vi "PH_gentec_M-Link.constructor.vi"(0 "name":string, 2 "data in":string, 5 "error in":errorcluster) -> (14 "i ref out":refnum<vi>, 16 "data out":string, 19 "error out":errorcluster)   [LabVIEW 2014, in "PH_gentec_M-Link.lvlib"]
doc: "This class is forseen to control a gentec-M-Link Energy- or Powermeter.\n\nThis class is part of the PHELIX device layer.\n\nauthor: Stefan Götte, GSI\n\nLicense Agreement for this software:\n\nCopyright (C)\nGesellschaft für Schwerionenforschung, GSI\nPlanckstr. 1\n64291 Darmstadt\nGermany\n\nContact: D.Beck@gsi.de \n\nThis program is free software; you can redistribute it and/or modify it under the terms of the \nGNU General Public License as published by the Free Software Foundation; either version 2 of \nthe license, or (at your option) any later version.\n\nThis program is distributed in the hope that it will be useful, but WITHOUT ANY WARRANTY; \nwithout even the implied warranty of MERCHANTABILITY or FITNESS FOR A PARTICULAR PURPOSE. See the GNU General License for more details (http://www.gnu.org).\n\nGesellschaft für Schwerionenforschung, GSI\nPlanckstr. 1, 64291 Darmstadt, Germany\nFor all questions and ideas contact: M.Richter@gsi.de, H.Brand@gsi.de or D.Beck@gsi.de.\nLast update: 16-JUN-2004"
uses:
  PH_gentec_M-Link.lvlib
  PH_Basics/PH_Powermeter_BaseClass/PH_Powermeter_BaseClass.State.ctl
  PH_Basics/PH_Class/PH_Class.lvlib
  PH_Basics/PH_Powermeter_BaseClass/PH_Powermeter_BaseClass.lvlib
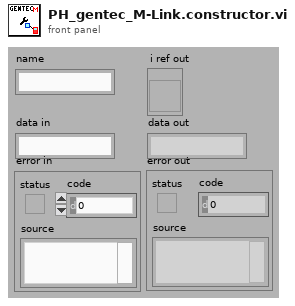
[diagram p1: front panel]
types:
  T1 = typedef "PH_Powermeter_BaseClass.lvlib/PH_Powermeter_BaseClass.State.ctl" = enum32{"off", "operating", "opened", "checked", "connected", "Sets to change", "running"}
  T2 = enum16{"SetAttribute", "GetAttribute", "CreateAttribute", "DestroyAttribute", "DestroyAllAtributes"}
  T3 = typedef "PH_gentec_M-Link.lvlib/PH_gentec_M-Link.i attribute.ctl" = cluster{"GUI References":cluster{"Wanted Head Settings":refnum<vi>, "Current Head Settings":refnum<vi>, "Set Auto Range":refnum<vi>, "Trigger Polarity":refnum<vi>, "Trigger Source":refnum<vi>, "Waveform Averages":refnum<vi>, "Continuous":refnum<vi>, "get one Value":refnum<vi>}, "Wanted Head Settings":T4, "Current Head Settings":T4}
  T4 = typedef "PH_gentec_M-Link.lvlib/PH_gentec_M-Link.Head Settings.ctl" = cluster{"Measurement Mode":T5, "Enable Anticipation":bool, "Set Auto Range":bool, "Block Signal":bool, "Set Head Attenuator":bool, "Enable SSE":bool, "Trigger Polarity":T6, "Trigger Source":T7, "Waveform Averages":T8, "Set Zero":i32, "Current":i32, "Start Data Flow":bool}
  T5 = typedef "gentec-M-Link - Driver.lvlib/gentec-M-Link.Measurement Mode.ctl" = u16
  T6 = typedef "gentec-M-Link - Driver.lvlib/gentec-M-Link.Trigger Polarity.ctl" = u16
  T7 = typedef "gentec-M-Link - Driver.lvlib/gentec-M-Link.Trigger Source.ctl" = u16
  T8 = typedef "gentec-M-Link - Driver.lvlib/gentec-M-Link.Waveform Averages.ctl" = u16
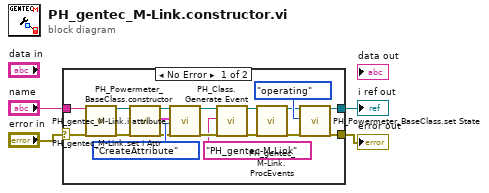
[diagram p0: block diagram]
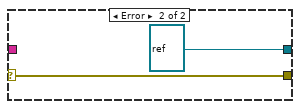
[diagram p2: hidden frame]
diagram:
  n1 = case shown="No Error" "error in" {
    selector: "error in" -> [w8 w24]
    tunnel: "name" -> [w9 _]
    tunnel: [w22 refnum<vi> refnum ("i ref out")] -> w3
    tunnel: [w21 w24] -> w2
    frame No Error {
      n2 = call "PH_Powermeter_BaseClass.constructor.vi"("name"=w9, "error in"=w8) -> ("i ref out"=w10:refnum<vi>, "error out"=w11:errorcluster)  [unwired: 15 in, 1 out]
      n3 = call "PH_gentec_M-Link.set i Attr.vi"("i ref in"=w10, "error in"=w11) -> ("i ref out"=w14:refnum<vi>, "i Attributes"=w12:T3, "error out"=w13:errorcluster)  [unwired: 15 in]
      n4 = call "PH_gentec_M-Link.i attribute.vi"("VI Refnum"=w14, "CLASS.i attribute"=w12, "Action"=T2."CreateAttribute", "error in (no error)"=w13) -> ("VI Refnum out"=w19:refnum<vi>, "error out"=w18:errorcluster)  [unwired: 13 in, 1 out]
      n5 = call "PH_Class.Generate Event.vi"("i ref in"=w19, "Class"="PH_gentec-M-Link", "error in (no error)"=w18) -> ("i ref out"=w16:refnum<vi>, "error out"=w15:errorcluster)  [unwired: 15 in]
      n6 = call "PH_gentec_M-Link.ProcEvents.vi"("i ref in"=w16, "error in"=w15) -> ("i ref out"=w6:refnum<vi>, "error out"=w5:errorcluster)  [unwired: 16 in]
      n7 = call "PH_Powermeter_BaseClass.set State.vi"("VI in"=w6, "State"=PH_Powermeter_BaseClass.State."operating", "error in (no error)"=w5) -> ("VI out"=w22:refnum<vi>, "error out"=w21:errorcluster)  [unwired: 15 in]
    }
    frame Error {
    }
  }
  "i ref out" <- w3
  "error out" <- w2
